vi "Open Last FITS Reference.vi"(8 "error in (no error)":errorcluster, 11 "Save Image in":refnum<class "Save Image.lvclass">) -> (0 "error out":errorcluster, 3 "Save Image out":refnum<class "Save Image.lvclass">)   [LabVIEW 2018, in "Save Image.lvclass"]
uses:
  Save Image.lvclass
  <userlib>/gfitsio/cfitsio-bitpix.ctl
  Save Image.lvclass/Save Image.ctl
  Interface/Interface.lvclass
  <userlib>/gfitsio/gfitsio.lvlib
  Simulated_Header/Simulated_Header.lvclass
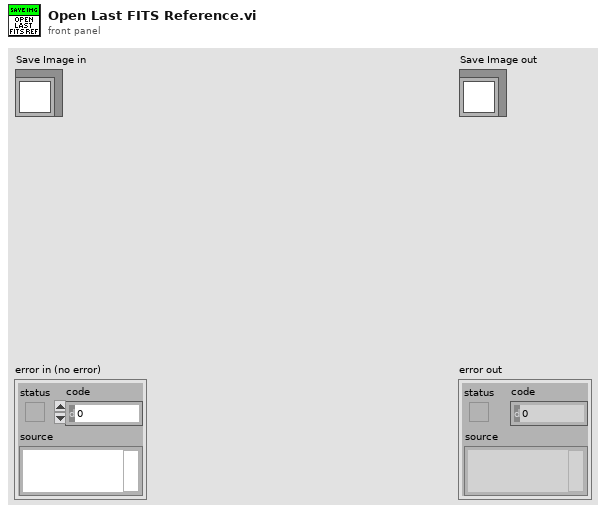
[diagram p1: front panel]
types:
  T1 = enum16{"open", "open or create", "create or replace", "create", "open (read only)"}
  T2 = enum16{"open", "open or create", "create", "create or replace"}
  T3 = typedef "gfitsio.lvlib/cfitsio-bitpix.ctl" = i32
  T4 = typedef "Shutter_mode typedef.ctl" = enum16{"Auto", "Open", "Close", "N/A (3)", "Open FVB Series", "Open Any Series"}
  T5 = typedef "ReadMode_mode typedef.ctl" = enum16{"Full Vertical Binning", "Multi-Track", "Random-Track", "Single-Track", "Image"}
  T6 = typedef "AcquisitionMode_mode typedef.ctl" = enum16{"Reserved (0)", "Single Scan", "Accumulate", "Kinetics", "Fast Kinetics", "Run Till Abort", "Reserved (6)", "Reserved (7)", "Reserved (8)", "Time Delayed Integration"}
  T7 = cluster{"EXPTIME":sgl, "PREAMP":enum16{"Gain 1", "Gain 2"}, "READOUT_RATE":enum16{"30 MHz", "20 MHz", "10 MHz", "1 MHz"}, "EM_GAIN":u16, "VBIN":u16, "INITIAL_LINE":u16, "INITIAL_COLUMN":u16, "FINAL_LINE":u16, "FINAL_COLUMN":u16, "#FRAMES":u32, "#CUBES":u32, "TRIGGER_MODE":enum16{"Internal", "External", "N/A", "N/A_1", "N/A_2", "N/A_3", "External Start"}, "HBIN":u16, "SHUTTER_TTL":enum16{"TTL Low", "TTL High"}, "SHUTTER_MODE":T4, "SHUTTER_OPENING_TIME":u16, "SHUTTER_CLOSING_TIME":u16, "VERTICAL_SHIFT_SPEED":u16, "READ_MODE":T5, "FRAME_TRANSFER":bool, "VERTICAL_CLOCK_VOLTAGE":enum16{"0", "+1", "+2", "+3", "+4"}, "ACQUISITION_MODE":T6, "AD_CHANNEL":u16, "EM_MODE":enum16{"Electron Multiplying", "Conventional"}}
  T8 = typedef "gfitsio.lvlib/gfitsio-refnum.ctl" = refnum<k1>
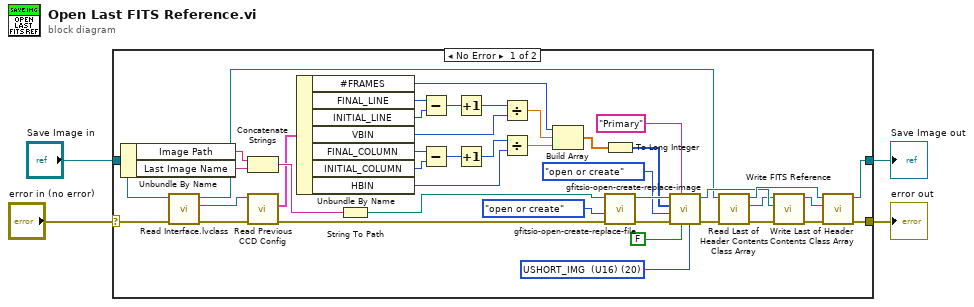
[diagram p0: block diagram]
diagram:
  n1 = case shown="No Error" "error in (no error)" {
    selector: "error in (no error)" -> [w7 w48]
    tunnel: [w12 w48] -> w3
    tunnel: [w19 w47] -> w1
    tunnel: "Save Image in" -> [w6 w47]
    frame No Error {
      w42 = T3 20 items=["<invalid type>"=0, "BYTE_IMG  (U8)"=8, "SHORT_IMG  (I16)"=16, "USHORT_IMG  (U16)"=20, "LONG_IMG  (I32)"=32, "ULONG_IMG  (U32)"=40, "FLOAT_IMG  (SGL)"=-32, "DOUBLE_IMG  (DBL)"=-64] ("image data type")
      n2 = Unbundle By Name(w6) -> ("Image Path"=w22:string, "Last Image Name"=w21:string)
      n3 = call "Read Interface.lvclass.vi"("error in (no error)"=w7, "Save Image in"=w6) -> ("error out"=w9:errorcluster, "Interface.lvclass"=w10:refnum<class "Interface.lvclass">, "Save Image out"=w5:refnum<class "Save Image.lvclass">)  [unwired: 7 in]
      n4 = Concatenate Strings(w22, w21) -> (w41:string)
      n5 = call "Read Previous CCD Config.vi"("error in (no error)"=w9, "Interface in"=w10) -> ("error out"=w8:errorcluster, "Previous CCD Config"=w11:T7)  [unwired: 7 in, 1 out]
      n6 = Unbundle By Name(w11) -> ("#FRAMES"=w23:u32, "FINAL_LINE"=w29:u16, "INITIAL_LINE"=w28:u16, "VBIN"=w27:u16, "FINAL_COLUMN"=w26:u16, "INITIAL_COLUMN"=w25:u16, "HBIN"=w24:u16)
      n7 = String To Path(string=w41) -> (path=w40:path)
      n8 = Subtract(x=w29, y=w28) -> (x-y=w36:u16)
      n9 = Subtract(x=w26, y=w25) -> (x-y=w37:u16)
      n10 = Increment(x=w36) -> (x+1=w35:u16)
      n11 = Increment(x=w37) -> (x+1=w34:u16)
      n12 = Divide(x=w35, y=w27) -> (x/y=w33:dbl)
      n13 = Divide(x=w34, y=w24) -> (x/y=w32:dbl)
      n14 = Build Array(w23, w33, w32) -> (w31:dbl[])
      n15 = To Long Integer(number=w31) -> (32bit integer=w30:i32[])
      n16 = call <userlib>:"gfitsio-open-create-replace-file.vi"("error in (no error)"=w8, "function (open)"=T1."open or create", "file path (dialog if empty)"=w40) -> ("error out"=w46:errorcluster, "gfits refnum"=w45:T8)  [unwired: 6 in, 1 out]
      n17 = call <userlib>:"gfitsio-open-create-replace-image.vi"("image data type"=w42, "advisory dialog? (display:T)"=FALSE, "hdu name (dialog if empty)"="Primary" ("prompt"), "error in (no error)"=w46, "function (create or replace)"=T2."open or create" ("function (open or create)"), "naxes"=w30, "gfits refnum"=w45) -> ("error out"=w13:errorcluster, "dup gfits refnum"=w18:T8)  [unwired: 2 in, 1 out]
      n18 = call "Read Last of Header Contents Class Array.vi"("error in (no error)"=w13, "Save Image in"=w5) -> ("error out"=w14:errorcluster, "Simulated_Header.lvclass"=w17:refnum<class "Simulated_Header.lvclass">, "Save Image out"=w20:refnum<class "Save Image.lvclass">)  [unwired: 7 in]
      n19 = call "Write FITS Reference.vi"("error in (no error)"=w14, "gfits refnum"=w18, "Simulated_Header in"=w17) -> ("error out"=w15:errorcluster, "Simulated_Header out"=w16:refnum<class "Simulated_Header.lvclass">)  [unwired: 7 in]
      n20 = call "Write Last of Header Contents Class Array.vi"("error in (no error)"=w15, "Simulated_Header.lvclass"=w16, "Save Image in"=w20) -> ("error out"=w12:errorcluster, "Save Image out"=w19:refnum<class "Save Image.lvclass">)  [unwired: 7 in]
    }
    frame Error {
    }
  }
  "error out" <- w3
  "Save Image out" <- w1
